vi "fgv_angle_vel_buffer.vi"(7 "agv_cmd_angle":enum16{"ini", "write", "read"}(ring), 9 "index":i32, 10 "angle_vel in":dbl, 11 "dim size":i32) -> (3 "angle_vel out":dbl)   [LabVIEW 2018]
uses:
  <vilib>/Analysis/baseanly.llb/Mean (DBL).vi
  <vilib>/Analysis/NI_AALBase.lvlib
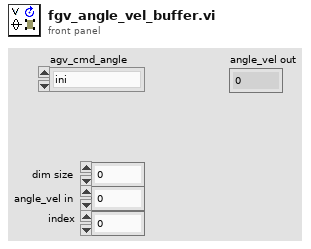
[diagram p1: front panel]
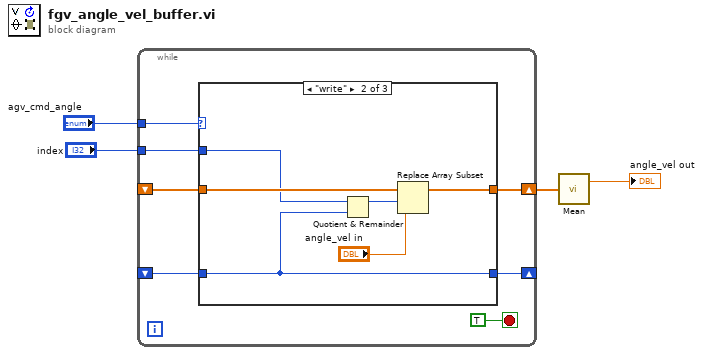
[diagram p0: block diagram]
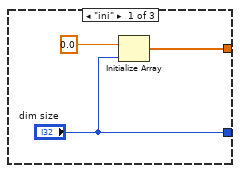
[diagram p2: hidden frame]
diagram:
  n1 = while {
    tunnel: "agv_cmd_angle" -> [w10]
    shift-right: [w9] -> w3
    shift-left: _ -> [w8]
    tunnel: "index" -> [w7]
    shift-right: [w6] -> _
    shift-left: _ -> [w5]
    stop <- TRUE stop-if-true
    n2 = case shown="\"write\"" w10 {
      tunnel: [w13 w19 w22] -> w9
      tunnel: w8 -> [_ w20 w22]
      tunnel: w7 -> [_ w16 _]
      tunnel: ["dim size" w15 w21] -> w6
      tunnel: w5 -> [_ w15 w21]
      frame "ini" {
        n3 = Initialize Array(0.0 ("원소"), "dim size") -> (w13:dbl[])
      }
      frame "write" {
        n4 = Quotient & Remainder(x=w16, y=w15) -> (x-y*floor(x/y)=w18:i32)  [unwired: 1 out]
        n5 = Replace Array Subset(array=w20, new element="angle_vel in", index=w18) -> (w19:dbl[])
      }
      frame "read", Default {
      }
    }
  }
  n6 = call-poly <vilib>:"Mean.vi"("X"=w3) -> ("mean"=→"angle_vel out":dbl)  [unwired: 1 out]
